vi "Get Config Log.vi"(7 "Parse Timestamp":string, 8 "error in (no error)":errorcluster, 10 "Parse All":bool, 11 "Plugin Manager in":refnum<class "CIFPluginManager.lvclass">) -> (0 "error out":errorcluster, 2 "Filtered Config Entries":string, 3 "Plugin Manager out":refnum<class "CIFPluginManager.lvclass">)   [LabVIEW 2021, in "CIFPluginManager.lvclass"]
uses:
  CIFPluginManager.lvclass
  CIFPluginManager.lvclass/CIFPluginManager.ctl
  <vilib>/CIF Foundation/CIF Core/CIFUtilities/CIFLogs/CIFLogs.lvlib
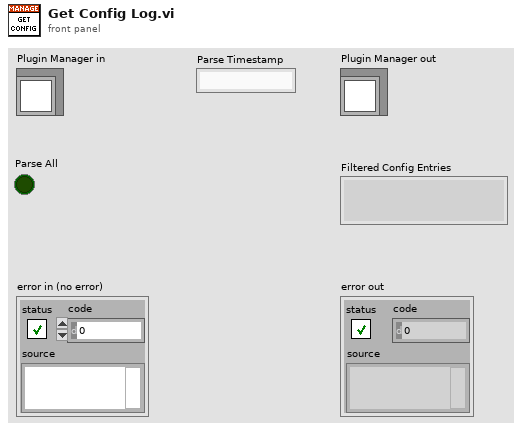
[diagram p1: front panel]
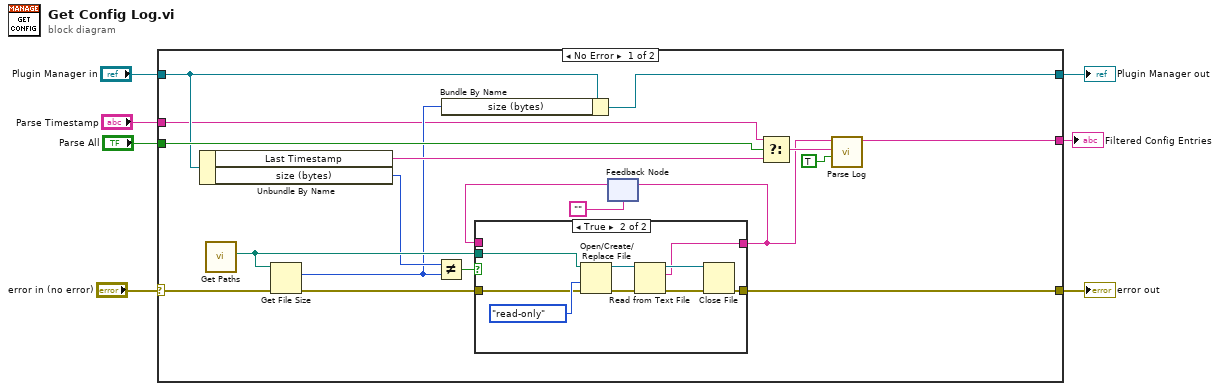
[diagram p0: block diagram]
diagram:
  n1 = case shown="No Error" "error in (no error)" {
    selector: "error in (no error)" -> [w19 w38]
    tunnel: [w25 w38] -> w6
    tunnel: [w10 w37] -> w4
    tunnel: "Plugin Manager in" -> [w11 w37]
    tunnel: [w22 _] -> w2
    tunnel: "Parse All" -> [w24 _]
    tunnel: "Parse Timestamp" -> [w8 _]
    frame No Error {
      n2 = Unbundle By Name(w11) -> ("Last Timestamp"=w12:string, "size (bytes)"=w17:i64)
      n3 = call <vilib>:"Get Paths.vi"() -> ("Config Log"=w20:path)  [unwired: 9 in, 2 out]
      n4 = Get File Size(file=w20, error in=w19) -> (size (in bytes)=w9:i64, 0:w18:errorcluster)  [unwired: 1 out]
      n5 = Not Equal?(x=w17, y=w9) -> (x != y?=w16:bool)
      n6 = Bundle By Name(cluster=w11, "size (bytes)"=w9) -> (w10:refnum<class "CIFPluginManager.lvclass">)
      n7 = feedback #1("") -> (w13:string)
      n8 = case shown="True" w16 {
        tunnel: [w26 w32] -> w25
        tunnel: w20 -> [_ w30]
        tunnel: w18 -> [w26 w29]
        tunnel: [w27 w28] -> w15
        tunnel: w13 -> [w27 _]
        frame False {
        }
        frame True {
          n9 = Open/Create/Replace File(file path (use dialog)=w30, error in=w29, access (0:read/write)=enum16{"read/write", "read-only", "write-only"}."read-only") -> (refnum out=w35:refnum<file>, error out=w34:errorcluster)  [unwired: 3 in, 1 out]
          n10 = Read from Text File(file (use dialog)=w35, error in=w34) -> (refnum out=w36:refnum<file>, text=w28:string, error out=w33:errorcluster)  [unwired: 2 in, 1 out]
          n11 = Close File(refnum=w36, error in=w33) -> (error out=w32:errorcluster)  [unwired: 1 out]
        }
      }
      n12 = feedback-in #1(w15) -> ()
      n13 = Select(t=w8, s=w24, f=w12) -> (s? t:f=w23:string)
      n14 = call <vilib>:"Parse Log.vi"("Strip Timestamp"=TRUE, "Index Timestamp"=w23, "Log"=w15) -> ("Filtered Config Entries"=w22:string)  [unwired: 8 in]
    }
    frame Error {
    }
  }
  "error out" <- w6
  "Plugin Manager out" <- w4
  "Filtered Config Entries" <- w2
